vi "Test Deserialize Boolean.vi"(8 "error in (no error)":errorcluster) -> (0 "error out":errorcluster)   [LabVIEW 2013]
uses:
  src/Deserializer/JSON Deserializer/JSON Deserializer.lvclass
  <vilib>/addons/_JKI Toolkits/Caraya/classes/Test/Test.lvclass
  <vilib>/addons/_JKI Toolkits/Caraya/classes/Assert/Assert.lvclass
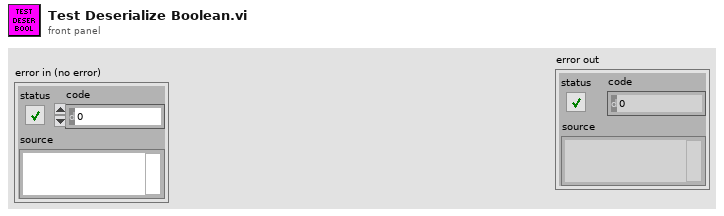
[diagram p1: front panel]
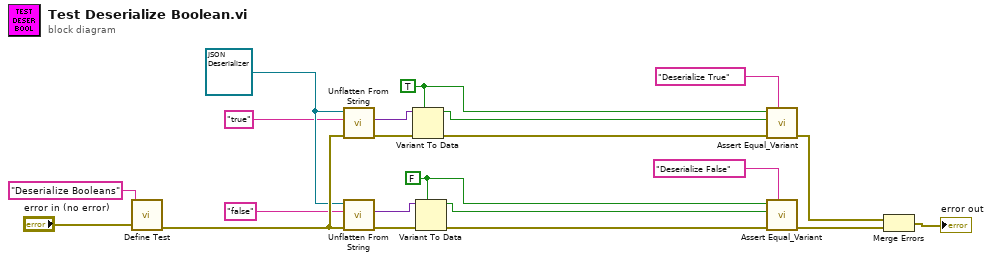
[diagram p0: block diagram]
diagram:
  w11 = refnum<class "JSON Deserializer.lvclass"> refnum ("JKI JSON Serialization.lvlib:JSON Deserializer.lvclass")
  w1 = TRUE
  w5 = FALSE
  n1 = call <vilib>:"Define Test.vi"("error in (no error)"="error in (no error)", "Label (VI Title)"="Deserialize Booleans") -> ("error out"=w16:errorcluster)  [unwired: 9 in]
  n2 = call-dynamic "Unflatten From String.vi"("error in (no error)"=w16, "String"="true", "Deserializer in"=w11) -> ("error out"=w18:errorcluster, "Variant"=w8:variant)  [unwired: 6 in, 1 out]
  n3 = call-dynamic "Unflatten From String.vi"("error in (no error)"=w16, "String"="false", "Deserializer in"=w11) -> ("error out"=w20:errorcluster, "Variant"=w6:variant)  [unwired: 6 in, 1 out]
  n4 = Variant To Data(error in=w18, type=w1, Variant=w8) -> (data=w2:bool, error out=w9:errorcluster)
  n5 = Variant To Data(error in=w20, type=w5, Variant=w6) -> (data=w3:bool, error out=w7:errorcluster)
  n6 = call <vilib>:"Assert Equal_Variant.vi"("Label"="Deserialize True", "error in (no error)"=w9, "Y"=w2, "X"=w1) -> ("error out"=w13:errorcluster)  [unwired: 7 in]
  n7 = call <vilib>:"Assert Equal_Variant.vi"("Label"="Deserialize False", "error in (no error)"=w7, "Y"=w3, "X"=w5) -> ("error out"=w14:errorcluster)  [unwired: 7 in]
  n8 = Merge Errors(w13, w14) -> (→"error out":errorcluster)
